vi "globals_ShootDualTalonSRX.vi"() -> ()   [LabVIEW 2019, in "ShootDualTalonSRX_Motor_Pair.lvlib"]
uses:
  ShootDualTalonSRX_Motor_Pair.lvlib
panel:
  out "Applied Output  L":dbl format="%.5f"
  out "Encoder Velocity Units Per 100ms L":dbl format="%.5f"
  out "Target Velocity Units per 100ms L":dbl format="%.5f"
  out "Raw encoder counts  L":dbl
  out "Speed Dmd FeedBack  FT/SEC L":dbl format="%.5f"
  out "Speed  FT/SEC L":dbl format="%.5f"
  out "Distance FT L":dbl format="%.5f"
  out "Applied Output R":dbl format="%.5f"
  out "Encoder Velocity Units Per 100ms R":dbl format="%.5f"
  out "Target Velocity Units per 100ms R":dbl format="%.5f"
  out "Raw encoder counts R":dbl
  out "Speed Dmd Feedback FT/SEC R":dbl format="%.5f"
  out "Speed FT/SEC R":dbl format="%.5f"
  out "Distance FT R":dbl format="%.5f"
  out "Drv_Right_Open_Loop_KF":dbl format="%.6f"
  out "Drv_Left_Open_Loop_KF":dbl format="%.6f"
  out "Drv_Right_Speed_Demand":dbl format="%.6f"
  out "Drv_Left_Speed_Demand":dbl format="%.6f"
  out "Drv_Speed_Ctrl_Enabled":bool
  out "Drv_Enc_Counts_Per_Rev":dbl=1440.0 format="%.6f"
  out "Drv_Wheel_Radius_Inches":dbl=3.0 format="%.6f"
  out "Drv_1_Over_Max_Speed_VELUNITS":dbl=0.1 format="%.6f"
  out "Drv_Max_Speed_VELUNITS":dbl=10.0 format="%.6f"
  out "Drv_Count_Per_VELUNITS_in_0_1_SEC":dbl format="%.6f"
  out "Drv_VELUNITS_Per_Count_in_0_1_SEC":dbl format="%.6f"
  out "Drv_DIST_Per_Count":dbl format="%.6f"
  out "Drv_Count_Per_DIST":dbl format="%.6f"
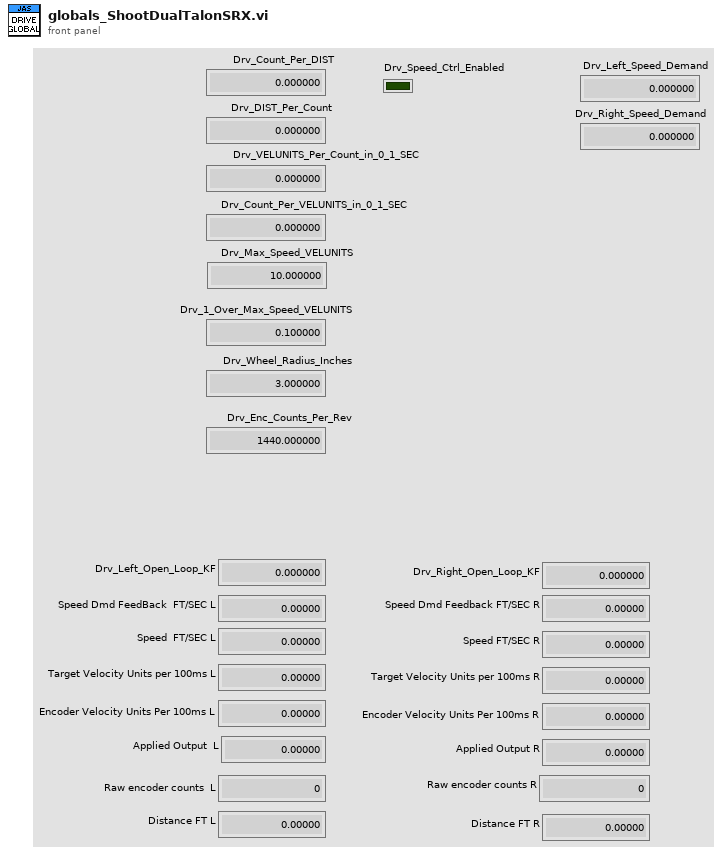
[diagram p1: front panel]
diagram:
